vi "XNET String To IO Name (Frame).vi"(3 "string":string) -> (0 "XNET Frame":refnum<k21>)   [LabVIEW 2018]
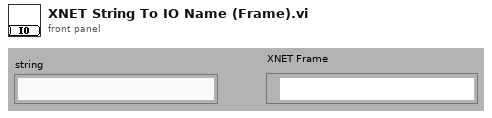
[diagram p1: front panel]
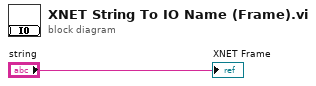
[diagram p0: block diagram]
diagram:
  "XNET Frame" <- "string"
